vi "AsignRequestToPersonnel.vi"(8 "error in (no error)":errorcluster, 11 "Request in":refnum<class "Request.lvclass">) -> (0 "error out":errorcluster)   [LabVIEW 2015]
uses:
  LVClasses/Request/Request.lvclass
  TypeDef/RequestActionEnum.ctl
  LVClasses/Request/Request.lvclass/Request.ctl
  TypeDef/PersonnelActions.ctl
  LVClasses/Request/Read Summary.vi
  LVClasses/Request/Read PersonnelType.vi
  LVClasses/Request/Read StartName.vi
  LVClasses/Request/Read Request Type.vi
  LVClasses/Request/Write PUID.vi
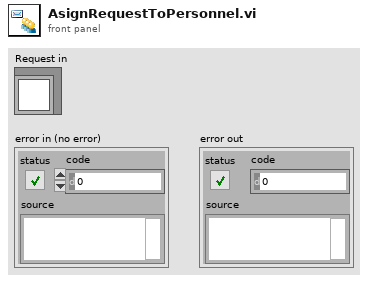
[diagram p1: front panel]
types:
  T1 = typedef "RequestActionEnum.ctl" = enum16{"Init", "ReadRequests", "ReadRequest", "AddRequest", "RemoveRequest", "ToDisk", "Ack", "Complete", "CheckAlarms", "PIntoRoom", "Read Summary", "GetRequestForRoom"}
  T2 = typedef "Request.lvclass/PersonnelType.ctl" = u16
  T3 = typedef "Request.lvclass/RequestType.ctl" = enum16{"Specific Call To Room", "General Call To Room"}
  T4 = typedef "PersonnelActions.ctl" = enum16{"Init", "Read Personnel", "Add Personnel", "Remove Personnel", "Read Name", "Write Name", "Read Role", "Write Role", "Read Requests", "Add Requests", "Remove Requests", "Read PUIDs", "Read PUIDs for Role"}
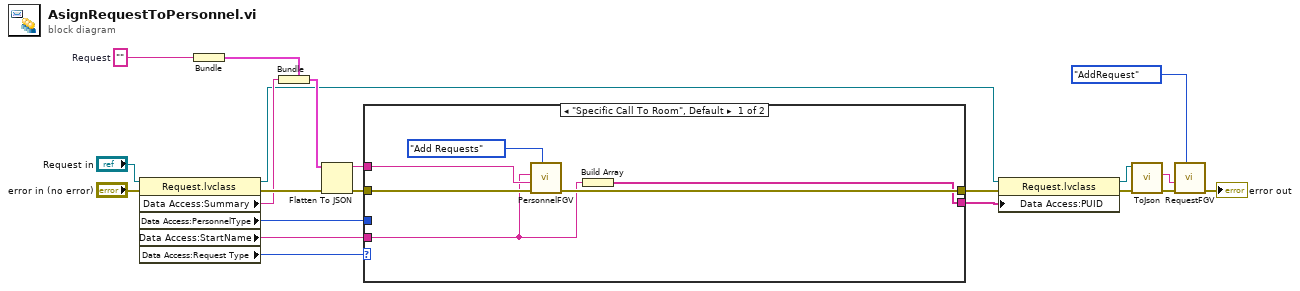
[diagram p0: block diagram]
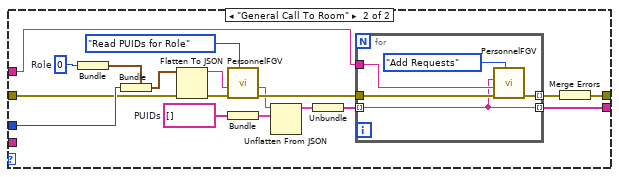
[diagram p2: hidden frame]
diagram:
  w14 = ""  # Request
  n1 = property class="Request.lvclass"(reference="Request in", error in="error in (no error)") -> (reference out=w7:refnum<class "Request.lvclass">, error out=w17:errorcluster, "Data Access:Summary"=w13:string, "Data Access:PersonnelType"=w18:T2, "Data Access:StartName"=w10:string, "Data Access:Request Type"=w20:T3)
  n2 = Bundle("Request"=w14) -> (w15:cluster{"Request":string})  [unwired: 1 in]
  n3 = Bundle(cluster=w15, "Request"=w13) -> (w12:cluster{"Request":string})
  n4 = Flatten To JSON(anything=w12, error in (no error)=w17) -> (JSON string=w11:string, 11:w16:errorcluster)  [unwired: 1 in]
  n5 = case shown="\"Specific Call To Room\", Default" w20 {
    tunnel: w10 -> [w22 _]
    tunnel: w16 -> [w25 w39]
    tunnel: [w26 w35] -> w1
    tunnel: w18 -> [_ w42]
    tunnel: w11 -> [w24 w29]
    tunnel: [w23 w28] -> w6
    frame "Specific Call To Room", Default {
      n6 = call "PersonnelFGV.vi"("Actions"=PersonnelActions."Add Requests", "error in (no error)"=w25, "Data In"=w24, "PUID"=w22) -> ("error out"=w26:errorcluster)  [unwired: 6 in, 1 out]
      n7 = Build Array(w22) -> (w23:string[])
    }
    frame "General Call To Room" {
      w34 = string[] []  # PUIDs
      w44 = 0  # Role
      n8 = Bundle("Role"=w44) -> (w40:cluster{"Role":i32})  [unwired: 1 in]
      n9 = Bundle(cluster=w40, "Role"=w42) -> (w41:cluster{"Role":i32})
      n10 = Flatten To JSON(anything=w41, error in (no error)=w39) -> (JSON string=w43:string, 11:w38:errorcluster)  [unwired: 1 in]
      n11 = call "PersonnelFGV.vi"("Actions"=PersonnelActions."Read PUIDs for Role", "error in (no error)"=w38, "Data In"=w43) -> ("error out"=w37:errorcluster, "Data Out"=w32:string)  [unwired: 7 in]
      n12 = Bundle("PUIDs"=w34) -> (w33:cluster{"PUIDs":string[]})  [unwired: 1 in]
      n13 = Unflatten From JSON(JSON string=w32, type and defaults=w33) -> (value=w31:cluster{"PUIDs":string[]})  [unwired: 5 in, 1 out]
      n14 = Unbundle(w31) -> ("PUIDs"=w30:string[])
      n15 = for {
        tunnel: w37 -> [w50]
        tunnel: [w49] -> w36 mode=indexing
        tunnel: w29 -> [w48]
        tunnel: w30 -> [w46] mode=indexing
        tunnel: [w46] -> w28 mode=indexing
        n16 = call "PersonnelFGV.vi"("Actions"=PersonnelActions."Add Requests", "error in (no error)"=w50, "Data In"=w48, "PUID"=w46) -> ("error out"=w49:errorcluster)  [unwired: 6 in, 1 out]
      }
      n17 = Merge Errors(w36) -> (w35:errorcluster)
    }
  }
  n18 = property class="Request.lvclass"(reference=w7, error in=w1, "Data Access:PUID"=w6) -> (reference out=w5:refnum<class "Request.lvclass">, error out=w2:errorcluster)
  n19 = call "ToJson.vi"("error in (no error)"=w2, "Request"=w5) -> ("error out"=w3:errorcluster, "Request"=w4:string)  [unwired: 8 in]
  n20 = call "RequestFGV.vi"("Actions"=RequestActionEnum."AddRequest", "error in (no error)"=w3, "Data In"=w4) -> ("error out"=→"error out":errorcluster)  [unwired: 7 in, 1 out]
